vi "input_fgv.vi"(1 "simulate":bool=TRUE, 2 "simulate input":bool=TRUE, 3 "Line(s)":tag="Dev8/port0/line0:7", 4 "input number":i32, 5 "action":T1) -> (0 "data out":bool[](array[boolean]))   [LabVIEW 2016]
uses:
  input.ctl
panel:
  out "simulate data":bool[](array[boolean])
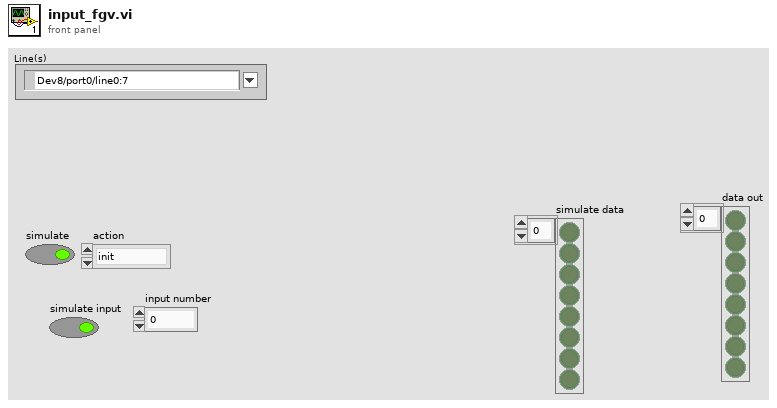
[diagram p1: front panel]
types:
  T1 = typedef "input.ctl" = enum16{"init", "read", "set_sim_val"}
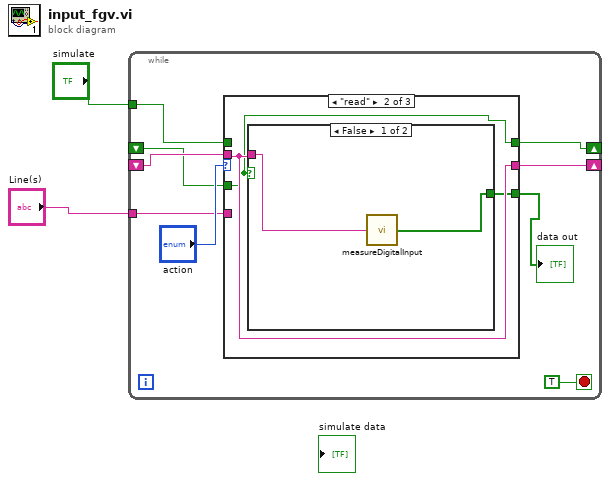
[diagram p0: block diagram]
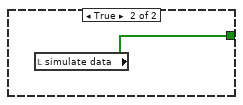
[diagram p3: hidden frame]
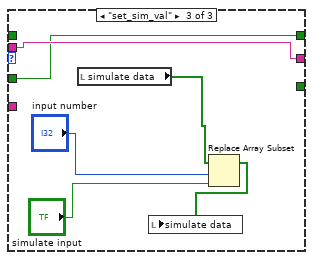
[diagram p4: hidden frame]
diagram:
  n1 = while {
    shift-right: [w9] -> _
    shift-left: _ -> [w7]
    tunnel: "Line(s)" -> [w8]
    shift-right: [w5] -> _
    shift-left: _ -> [w6]
    tunnel: "simulate" -> [w4]
    stop <- TRUE stop-if-true
    n2 = case shown="\"read\"" "action" {
      tunnel: [w13 w16 w25] -> w9
      tunnel: w8 -> [w13 _ _]
      tunnel: w7 -> [_ w16 w25]
      tunnel: w6 -> [_ w14 w21]
      tunnel: [_ w15 _] -> w3
      tunnel: [w12 w14 w21] -> w5
      tunnel: w4 -> [w12 _ _]
      frame "init", Default {
      }
      frame "read" {
        n3 = case shown="False" w14 {
          tunnel: w16 -> [w17 _]
          tunnel: [w18 w19] -> w15
          frame False {
            n4 = call "measureDigitalInput.vi"("Line(s)"=w17) -> ("data"=w18:bool[])
          }
          frame True {
            n5 = local read "simulate data"() -> (w19:bool[])
          }
        }
      }
      frame "set_sim_val" {
        n6 = local read "simulate data"() -> (w24:bool[])
        n7 = Replace Array Subset(array=w24, new element="simulate input", index="input number") -> (w22:bool[])
        n8 = local write "simulate data"(w22) -> ()
      }
    }
    "data out" <- w3
  }
